vi "Get_Data.vi"(8 "error in (no error)":errorcluster caption="entrée d'erreur (pas d'erreur)", 11 "Firebase Benches en entrée":refnum<class "Firebase Benches.lvclass">) -> (0 "error out":errorcluster caption="sortie d'erreur", 3 "Firebase Benches en sortie":refnum<class "Firebase Benches.lvclass">)   [LabVIEW 2020, in "Library Instrument & Equipement.lvlib" / "Library FireBase.lvlib" / "Firebase Benches.lvclass"]
doc: "Returns all data Use Nb_To_Read to determine the number to read\nPlease initialise the following values\n - Name BDD\n - Document\n - API Key\n - Nb To Read"
uses:
  Firebase Benches.lvclass
  C:/Users/ngarcin/OneDrive - Altyor/Standard TB/Class/Firebase/Source/Firebase Altyor/Firebase Altyor.lvclass
  C:/Users/ngarcin/OneDrive - Altyor/Standard TB/Class/Firebase/Source/Firebase Driver/Firebase Driver.lvclass
  Firebase Benches.lvclass/Firebase Benches.ctl
  JSON API/JSON Value/Set from JSON string.vi
  JSON API/JSON Value/JSON Value.lvclass
  Firebase Altyor/Firebase Altyor.lvclass
  JSON API/Variant JSON/Variant JSON.lvlib
  JSON API/Get Polymorphic/JSON GetSet.lvlib
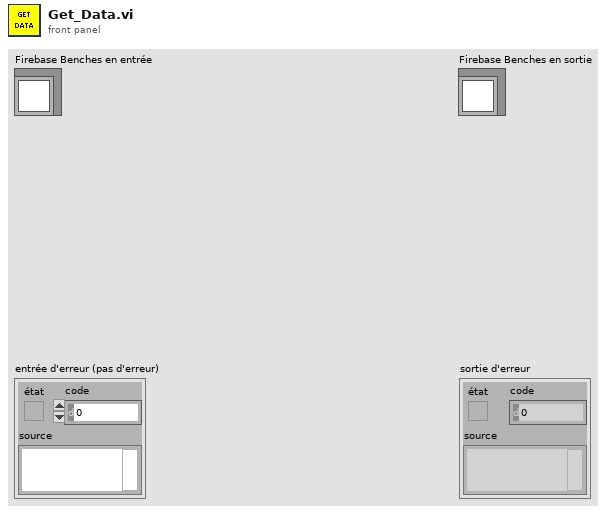
[diagram p1: front panel]
types:
  T1 = cluster{"name":string, "fields":cluster{"Result":cluster{"booleanValue":bool}, "CreationDate":cluster{"timestampValue":string}, "Batch":cluster{"stringValue":string}, "SerialNumber":cluster{"stringValue":string}, "EndOfProduction":cluster{"timestampValue":string}, "FW_Version":cluster{"mapValue":cluster{"fields":cluster{"Bootloader":cluster{"mapValue":cluster{"fields":cluster{"File_Name":cluster{"stringValue":string}, "Version":cluster{"mapValue":cluster{"fields":cluster{"Major":cluster{"stringValue":string}, "Minor":cluster{"stringValue":string}}}}, "Checksum":cluster{"stringValue":string}}}}, "SoftDevice":cluster{"mapValue":cluster{"fields":cluster{"File_Name":cluster{"stringValue":string}, "Version":cluster{"mapValue":cluster{"fields":cluster{"Major":cluster{"stringValue":string}, "Minor":cluster{"stringValue":string}}}}, "Checksum":cluster{"stringValue":string}}}}, "DFU":cluster{"mapValue":cluster{"fields":cluster{"File_Name":cluster{"stringValue":string}, "Version":cluster{"mapValue":cluster{"fields":cluster{"Major":cluster{"stringValue":string}, "Minor":cluster{"stringValue":string}}}}, "Checksum":cluster{"stringValue":string}}}}}}}, "PartNumber":cluster{"stringValue":string}, "OrderNumber":cluster{"stringValue":string}, "Operator":cluster{"stringValue":string}}}[]
  T2 = cluster{"documents":cluster{"name":string, "fields":cluster{"Result":cluster{"booleanValue":bool}, "CreationDate":cluster{"timestampValue":string}, "Batch":cluster{"stringValue":string}, "SerialNumber":cluster{"stringValue":string}, "EndOfProduction":cluster{"timestampValue":string}, "FW_Version":cluster{"mapValue":cluster{"fields":cluster{"Bootloader":cluster{"mapValue":cluster{"fields":cluster{"File_Name":cluster{"stringValue":string}, "Version":cluster{"mapValue":cluster{"fields":cluster{"Major":cluster{"stringValue":string}, "Minor":cluster{"stringValue":string}}}}, "Checksum":cluster{"stringValue":string}}}}, "SoftDevice":cluster{"mapValue":cluster{"fields":cluster{"File_Name":cluster{"stringValue":string}, "Version":cluster{"mapValue":cluster{"fields":cluster{"Major":cluster{"stringValue":string}, "Minor":cluster{"stringValue":string}}}}, "Checksum":cluster{"stringValue":string}}}}, "DFU":cluster{"mapValue":cluster{"fields":cluster{"File_Name":cluster{"stringValue":string}, "Version":cluster{"mapValue":cluster{"fields":cluster{"Major":cluster{"stringValue":string}, "Minor":cluster{"stringValue":string}}}}, "Checksum":cluster{"stringValue":string}}}}}}}, "PartNumber":cluster{"stringValue":string}, "OrderNumber":cluster{"stringValue":string}, "Operator":cluster{"stringValue":string}}}[], "nextPageToken":string}
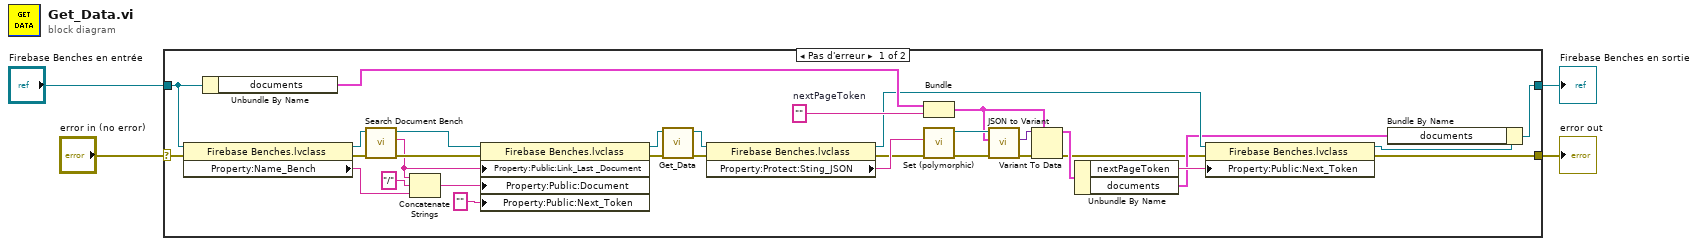
[diagram p0: block diagram]
diagram:
  n1 = case shown="Pas d'erreur" "error in (no error)" {
    selector: "error in (no error)" -> [w10 w38]
    tunnel: [w14 w37] -> w4
    tunnel: "Firebase Benches en entrée" -> [w9 w37]
    tunnel: [w11 w38] -> w2
    frame No Error {
      w23 = ""  # nextPageToken
      n2 = property class="Firebase Benches.lvclass"(reference=w9, error in=w10) -> (reference out=w8:refnum<class "Firebase Benches.lvclass">, error out=w7:errorcluster, "Property:Name_Bench"=w6:string)
      n3 = Unbundle By Name(w9) -> ("documents"=w22:T1)
      n4 = call "Search Document Bench.vi"("entrée d'erreur (pas d'erreur)"=w7, "Firebase Altyor en entrée"=w8) -> ("sortie d'erreur"=w36:errorcluster, "Source"=w34:string, "Firebase Altyor en sortie"=w35:refnum<class "Firebase Benches.lvclass">)  [unwired: 7 in]
      n5 = Concatenate Strings(w34, "/" ("chaîne"), w6) -> (w33:string)
      n6 = property class="Firebase Benches.lvclass"(reference=w35, error in=w36, "Property:Public:Link_Last _Document"=w34, "Property:Public:Document"=w33, "Property:Public:Next_Token"="" ("Next_Token")) -> (reference out=w30:refnum<class "Firebase Benches.lvclass">, error out=w29:errorcluster)
      n7 = call-parent "Get_Data.vi"("error in (no error)"=w29, "Firebase Altyor en entrée"=w30) -> ("error out"=w16:errorcluster, "Firebase Altyor en sortie"=w15:refnum<class "Firebase Benches.lvclass">)  [unwired: 8 in]
      n8 = property class="Firebase Benches.lvclass"(reference=w15, error in=w16) -> (reference out=w20:refnum<class "Firebase Benches.lvclass">, error out=w13:errorcluster, "Property:Protect:Sting_JSON"=w25:string)
      n9 = Bundle("documents"=w22, "nextPageToken"=w23) -> (w21:T2)  [unwired: 1 in]
      n10 = call-poly "Set (polymorphic).vi"("error in (no error)"=w13, "JSON stream"=w25) -> ("error out"=w26:errorcluster, "JSON Value out"=w28:refnum<class "JSON Value.lvclass">)  [unwired: 7 in, 1 out]
      n11 = call "JSON to Variant.vi"("error in (no error)"=w26, "Variant (Data Type)"=w21, "JSON Value"=w28) -> ("error out"=w27:errorcluster, "Variant out"=w5:variant)  [unwired: 7 in]
      n12 = Variant To Data(error in=w27, type=w21, Variant=w5) -> (data=w24:T2, error out=w12:errorcluster)
      n13 = Unbundle By Name(w24) -> ("nextPageToken"=w19:string, "documents"=w17:T1)
      n14 = property class="Firebase Benches.lvclass"(reference=w20, error in=w12, "Property:Public:Next_Token"=w19) -> (reference out=w18:refnum<class "Firebase Benches.lvclass">, error out=w11:errorcluster)
      n15 = Bundle By Name(cluster=w18, "documents"=w17) -> (w14:refnum<class "Firebase Benches.lvclass">)
    }
    frame Error {
    }
  }
  "Firebase Benches en sortie" <- w4
  "error out" <- w2
